vi "Stop Core.vi"(10 "final error code":i32, 11 "Device DDS Communications in":refnum<class "Device DDS Communications.lvclass">) -> (3 "Device DDS Communications out":refnum<class "Device DDS Communications.lvclass">)   [LabVIEW 2018, in "Device DDS Communications Framework.lvlib" / "Device DDS Communications.lvclass"]
doc: "(<B>Filename</B>: Actor Framework.lvlib:Actor.lvclass:Stop Core.vi)\n\nDefines what the actor does before it stops. Use the <B>final error code</B> input to determine whether the actor shut down in response to an error.\n\nBy default, this method does nothing. A descendant class may override it to define behavior, such as shutting down any processes the actor initiated in its override of the Actor Core method."
uses:
  Device DDS Communications.lvclass
  Device DDS Communications.lvclass/Device DDS Communications.ctl
  Device Communication and Control Abstract Actor/Device Communication and Control Abstract/Device Communication and Control Abstract.lvclass
  <vilib>/ORNL/CSEISMIC DDS/DDS Writer/DDS Writer.lvclass
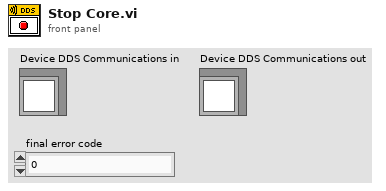
[diagram p1: front panel]
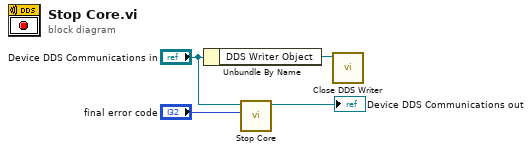
[diagram p0: block diagram]
diagram:
  n1 = Unbundle By Name("Device DDS Communications in") -> ("DDS Writer Object"=w1:refnum<class "DDS Writer.lvclass">)
  n2 = call-parent "Stop Core.vi"("final error code"="final error code", "EMS Generic in"="Device DDS Communications in") -> ("EMS Generic out"=→"Device DDS Communications out":refnum<class "Device DDS Communications.lvclass">)  [unwired: 9 in]
  n3 = call <vilib>:"Close DDS Writer.vi"("DDS Writer in"=w1) -> ()  [unwired: 10 in, 1 out]
